vi "TLMotorStartCtrl.vi"(4 "Error In (No Error)":errorcluster, 6 "SerialNum":i32, 7 "Motor Ref":refnum<k7>) -> (0 "Error Out":errorcluster, 3 "Motor Ref":refnum<k7>)   [LabVIEW 2014]
doc: "Starts the Motor control.\n\nIn\nMotor Ref - Reference to Motor control object.\nError In (No Error) - Standard LabView error cluster.\n\nOut\nMotor Ref - Reference to Motor control object.\nError Out - Standard LabView error cluster."
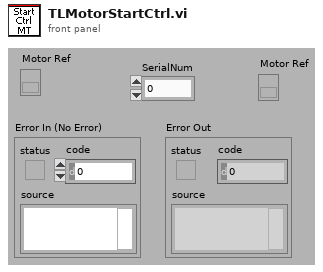
[diagram p1: front panel]
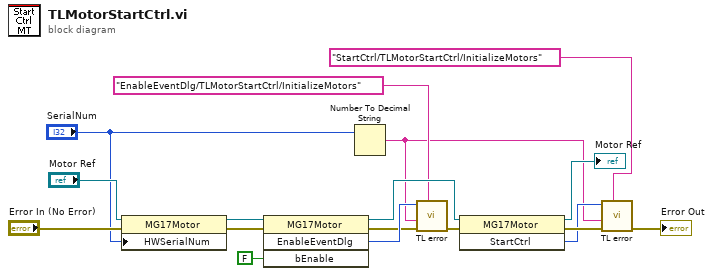
[diagram p0: block diagram]
diagram:
  n1 = property class="MG17Motor"(reference="Motor Ref", error in="Error In (No Error)", "HWSerialNum"="SerialNum") -> (reference out=w9:refnum<k7>, error out=w7:errorcluster)
  n2 = invoke class="MG17Motor" method="EnableEventDlg"(reference=w9, error in=w7, "bEnable"=FALSE) -> (reference out=w8:refnum<k7>, error out=w6:errorcluster, "EnableEventDlg"=w10:i32)  [unwired: 1 in, 1 out]
  n3 = Number To Decimal String(number="SerialNum") -> (decimal integer string=w2:string)  [unwired: 1 in]
  n4 = call "TL error.vi"("Input string"="EnableEventDlg/TLMotorStartCtrl/InitializeMotors", "error in (no error)"=w6, "Serial number of motor"=w2, "Return Code"=w10) -> ("error out"=w5:errorcluster)  [unwired: 7 in]
  n5 = invoke class="MG17Motor" method="StartCtrl"(reference=w8, error in=w5) -> (reference out=→"Motor Ref":refnum<k7>, error out=w17:errorcluster, "StartCtrl"=w16:i32)  [unwired: 1 in]
  n6 = call "TL error.vi"("Input string"="StartCtrl/TLMotorStartCtrl/InitializeMotors", "error in (no error)"=w17, "Serial number of motor"=w2, "Return Code"=w16) -> ("error out"=→"Error Out":errorcluster)  [unwired: 7 in]
